vi "HFRR ADV v02.vi"() -> ()   [LabVIEW 2025] (continued)
        n289 = event-data() -> ()  [unwired: 1 in, 6 out]
        n290 = local read "Calibration"() -> (w387:bool)
        n291 = case shown="False" w387 {
          frame False {
            n292 = property on="Calibration 2" class="TabCtl (strict)"("Visible"=FALSE) -> ()  [unwired: 2 in, 2 out]
            n293 = local write "Cal Password"("" ("Cal Password")) -> ()
          }
          frame True {
            n294 = property on="Calibration 2" class="TabCtl (strict)"("Visible"=TRUE) -> ()  [unwired: 2 in, 2 out]
            n295 = local write "Cal Password"("" ("Cal Password")) -> ()
          }
        }
        n296 = property on="Wrong Password" class="Str"("Visible"=FALSE) -> ()  [unwired: 2 in, 2 out]
      }
      event "Cal Password": Value Change {
        n297 = event-data() -> ()  [unwired: 1 in, 6 out]
        n298 = local read "Cal Password"() -> (w395:string)
        n299 = call <vilib>:"Trim Whitespace.vi"("string"=w395) -> ("trimmed string"=w394:string)  [unwired: 1 in]
        n300 = Equal?(x=w394, y="Cal@321") -> (x = y?=w392:bool)
        n301 = case shown="True" w392 {
          frame False {
            n302 = property on="Wrong Password" class="Str"("Visible"=TRUE) -> ()  [unwired: 2 in, 2 out]
          }
          frame True {
            n303 = property on="Wrong Password" class="Str"("Visible"=FALSE) -> ()  [unwired: 2 in, 2 out]
            n304 = local write "Main Tab"(T2."About" ("Main Tab")) -> ()
            n305 = local write "Cal Password"("" ("Cal Password")) -> ()
            n306 = local write "Main Dashboard Buttons"(T1."About" ("Main Dashboard Buttons")) -> ()
            n307 = local write "Tab Control 5"(T7."Temperature Calibration" ("Tab Control 5")) -> ()
            n308 = property on="Calibration 2" class="TabCtl (strict)"("Visible"=FALSE) -> ()  [unwired: 2 in, 2 out]
            n309 = property on="Tab Control 5" class="TabCtl (strict)"("Tabs Visible?"=FALSE ("Page Labels Display Visible?")) -> ()  [unwired: 2 in, 2 out]
            n310 = local write "Calibration"(FALSE ("Calibration")) -> ()
          }
        }
      }
      event "Quit": Value Change {
        n311 = event-data() -> ()  [unwired: 1 in, 6 out]
      }
    }
    n312 = Wait (ms)(milliseconds to wait=u32 100) -> ()  [unwired: 1 out]
  }
  n313 = local write "Auto stop temp"(w12) -> ()
  n314 = local write "main tab sub"(enum32{"Page 1", "Page 2"}."Page 1" ("main tab sub")) -> ()
  n315 = local write "USERNAME"(w31) -> ()
  n316 = local write "Main Tab"(T2."HOME" ("Main Tab")) -> ()
  n317 = local write "USER ID"(w31) -> ()
  n318 = property on="Auto Scar Check  2" class="Clust (strict)"("Visible"=w12) -> (error out=w16:errorcluster)  [unwired: 2 in, 1 out]
  n319 = property on="Quit" class="Bool (strict)"("Value"=FALSE ("Quit")) -> (error out=w33:errorcluster)  [unwired: 2 in, 1 out]
  n320 = while {
    shift-right: [w407] -> _
    shift-left: "Enum - Selector" -> [w408]
    stop <- w409 stop-if-true
    # "Auto Start Logic Loop"
    n321 = case shown="\"close\"" w408 {
      tunnel: [w412 w418 w429 w461 w492 Auto_Start_enum."Exit" ("Enum - Selector") Auto_Start_enum."Init" ("Enum - Selector")] -> w407
      frame "Init", Default {
        n322 = local read "Auto Start Test"() -> (w411:bool)
        n323 = Select(t=Auto_Start_enum."Humidity & Temperature On" ("Enum - Selector"), s=w411, f=Auto_Start_enum."Init") -> (s? t:f=w412:T10)
      }
      frame "Humidity & Temperature On" {
        n324 = flat-sequence {
          tunnel: [Auto_Start_enum."Reach point" ("Enum - Selector")] -> w415
          frame #0 {
            w419 = T13."Disabled and Grayed Out" ("Disabled")
            w420 = TRUE ("Heater Button")
            n325 = property on="Humidity" class="Bool (strict)"("DisabledEnum"=w419) -> ()  [unwired: 2 in, 2 out]
            n326 = property on="Heater Button" class="Bool (strict)"("DisabledEnum"=w419) -> ()  [unwired: 2 in, 2 out]
            n327 = local write "Heater Button"(w420) -> ()
            n328 = local write "Humidity"(w420) -> ()
          }
          frame #1 {
            n329 = Wait (ms)(milliseconds to wait=u32 1000) -> ()  [unwired: 1 out]
          }
          frame #2 {
            w422 = TRUE ("Reach point temp")
            n330 = local write "Reach point Humidity"(w422) -> ()
            n331 = local write "Reach point temp"(w422) -> ()
          }
        }
        n332 = local read "Auto Start Test"() -> (w417:bool)
        n333 = Not(x=w417) -> (.not. x?=w416:bool)
        n334 = Select(t=Auto_Start_enum."close", s=w416, f=w415) -> (s? t:f=w418:T10)
      }
      frame "Reach point" {
        w430 = TRUE ("PAUSE")
        w438 = 1.0 ("y")
        w441 = 1.0 ("y")
        n335 = local read "Set Temperature:"() -> (w442:dbl)
        n336 = local read "Set Humidity:"() -> (w437:dbl)
        n337 = local read "Humidity ( %RH )"() -> (w443:dbl)
        n338 = Add(x=w442, y=w441) -> (x+y=w440:dbl)
        n339 = Subtract(x=w442, y=w441) -> (x-y=w439:dbl)
        n340 = Add(x=w437, y=w438) -> (x+y=w436:dbl)
        n341 = Subtract(x=w437, y=w438) -> (x-y=w435:dbl)
        n342 = local read "TEMP"() -> (w444:dbl)
        n343 = In Range and Coerce(upper limit=w436, x=w443, lower limit=w435) -> (In Range?=w424:bool)  [unwired: 1 out]
        n344 = In Range and Coerce(upper limit=w440, x=w444, lower limit=w439) -> (In Range?=w425:bool)  [unwired: 1 out]
        n345 = case shown="True" w424 {
          frame False {
          }
          frame True {
            n346 = case shown="True" "Reach point Humidity" {
              selector: "Reach point Humidity" -> [_ w450]
              frame False {
              }
              frame True {
                n347 = local read "EVENT LOG"() -> (w447:string)
                n348 = Not(x=w450) -> (.not. x?=w449:bool)
                n349 = local write "Reach point Humidity"(w449) -> ()
                n350 = call "Event Log.vi"("Content"="Target Humidity reached", "EVENT LOG"=w447) -> ("EVENT LOG"=w448:string)  [unwired: 8 in, 1 out]
                n351 = local write "EVENT LOG"(w448) -> ()
              }
            }
          }
        }
        n352 = case shown="True" w425 {
          frame False {
          }
          frame True {
            n353 = case shown="True" "Reach point temp" {
              selector: "Reach point temp" -> [_ w456]
              frame False {
              }
              frame True {
                n354 = local read "EVENT LOG"() -> (w453:string)
                n355 = Not(x=w456) -> (.not. x?=w455:bool)
                n356 = local write "Reach point temp"(w455) -> ()
                n357 = call "Event Log.vi"("Content"="Target Temperature reached", "EVENT LOG"=w453) -> ("EVENT LOG"=w454:string)  [unwired: 8 in, 1 out]
                n358 = local write "EVENT LOG"(w454) -> ()
              }
            }
          }
        }
        n359 = local read "Auto Start Test"() -> (w428:bool)
        n360 = And(x=w425, y=w424) -> (x .and. y?=w434:bool)
        n361 = Select(t=Auto_Start_enum."Maintain Stage" ("Enum - Selector"), s=w434, f=Auto_Start_enum."Reach point" ("Enum - Selector")) -> (s? t:f=w431:T10)
        n362 = Not(x=w428) -> (.not. x?=w427:bool)
        n363 = Select(t=Auto_Start_enum."close", s=w427, f=w431) -> (s? t:f=w429:T10)
        n364 = call "ELAPSED TIMER VI.vi"("RESET"=w430, "PAUSE"=w430) -> ()  [unwired: 7 in, 3 out]
      }
      frame "Maintain Stage" {
        w470 = 2.0 ("y")
        w469 = 1.0 ("y")
        # "Humidity and  temperatures Set Point  have been reached"
        n365 = local read "Set Temperature:"() -> (w476:dbl)
        n366 = local read "Set Humidity:"() -> (w473:dbl)
        n367 = local read "Humidity ( %RH )"() -> (w477:dbl)
        n368 = Add(x=w476, y=w469) -> (x+y=w475:dbl)
        n369 = Subtract(x=w476, y=w469) -> (x-y=w474:dbl)
        n370 = local read "TEMP"() -> (w478:dbl)
        n371 = Add(x=w473, y=w470) -> (x+y=w472:dbl)
        n372 = Subtract(x=w473, y=w470) -> (x-y=w471:dbl)
        n373 = In Range and Coerce(upper limit=w475, x=w478, lower limit=w474) -> (In Range?=w468:bool)  [unwired: 1 out]
        n374 = In Range and Coerce(upper limit=w472, x=w477, lower limit=w471) -> (In Range?=w467:bool)  [unwired: 1 out]
        n375 = And(x=w468, y=w467) -> (x .and. y?=w466:bool)
        n376 = Not(x=w466) -> (.not. x?=w465:bool)
        n377 = call "ELAPSED TIMER VI.vi"("TARGET"=60.0, "RESET"=w465, "PAUSE"=FALSE) -> ("ELAPSED INDICATION"=w462:bool)  [unwired: 6 in, 2 out]
        n378 = case shown="True" w462 {
          tunnel: w462 -> [_ w481]
          tunnel: [Auto_Start_enum."Maintain Stage" ("Enum - Selector") w480] -> w460
          frame False {
          }
          frame True {
            n379 = stacked-sequence {
              tunnel: w481 -> [_ _ _ _ _]
              tunnel: [_ _ _ _ Auto_Start_enum."Start Stage" ("Enum - Selector")] -> w480
              frame #0 {
                n380 = local read "EVENT LOG"() -> (w483:string)
                n381 = call "Event Log.vi"("Content"="Humidity and temperature set point has stabilized.", "EVENT LOG"=w483) -> ("EVENT LOG"=w484:string)  [unwired: 8 in, 1 out]
                n382 = local write "EVENT LOG"(w484) -> ()
              }
              frame #1 {
                n383 = Wait (ms)(milliseconds to wait=u32 100) -> ()  [unwired: 1 out]
              }
              frame #2 {
                n384 = local read "EVENT LOG"() -> (w487:string)
                n385 = call "Event Log.vi"("Content"="Auto Test Started", "EVENT LOG"=w487) -> ("EVENT LOG"=w488:string)  [unwired: 8 in, 1 out]
                n386 = local write "EVENT LOG"(w488) -> ()
              }
              frame #3 {
                w489 = TRUE ("RUN")
                n387 = local write "RUN"(w489) -> ()
                "Auto Start Temp" <- w489
              }
              frame #4 {
              }
            }
          }
        }
        n388 = local read "Auto Start Test"() -> (w459:bool)
        n389 = Not(x=w459) -> (.not. x?=w458:bool)
        n390 = Select(t=Auto_Start_enum."close", s=w458, f=w460) -> (s? t:f=w461:T10)
      }
      frame "Start Stage" {
        w491 = TRUE ("PAUSE")
        n391 = local read "Auto Start Test"() -> (w496:bool)
        n392 = Not(x=w496) -> (.not. x?=w495:bool)
        n393 = Select(t=Auto_Start_enum."close" ("Enum - Selector"), s=w495, f=Auto_Start_enum."Start Stage" ("Enum - Selector")) -> (s? t:f=w492:T10)
        n394 = call "ELAPSED TIMER VI.vi"("RESET"=w491, "PAUSE"=w491) -> ()  [unwired: 7 in, 3 out]
      }
      frame "close" {
        w497 = FALSE ("Heater Button")
        n395 = local write "RUN"(w497) -> ()
        n396 = local write "Heater Button"(w497) -> ()
        n397 = local write "Humidity"(w497) -> ()
        n398 = local write "Auto Start Test"(w497) -> ()
      }
      frame "Exit" {
      }
    }
    n399 = Wait (ms)(milliseconds to wait=u32 100) -> ()  [unwired: 1 out]
    n400 = local read "Quit"() -> (w409:bool)
  }
  n401 = while {
    stop <- w526 stop-if-true
    w509 = errorcluster {"status"=FALSE, "code"=0, "source"=""} ("error in (no error) 3")
    # "this loop is for manual report generation"
    n402 = local read "Confirm Measrurement"() -> (w508:bool)
    n403 = case shown="True" w508 {
      selector: w508 -> [_ w616]
      tunnel: errorcluster {"status"=FALSE, "code"=0, "source"=""} ("error in (no error) 3") -> [_ w617]
      tunnel: [_ w615] -> _
      frame False {
      }
      frame True {
        n404 = stacked-sequence {
          tunnel: w617 -> [_ w650 _]
          tunnel: w616 -> [_ _ w757]
          tunnel: [_ w638 _] -> w615
          frame #0 {
            n405 = String To Path(string="C:\\LAB-IQ\\Image Calibrate v01.dcf") -> (path=w620:path)
            n406 = Open/Create/Replace File ("Open File")(file path (use dialog)=w620) -> (refnum out=w621:refnum<file>)  [unwired: 5 in, 2 out]
            n407 = for {
              N: 4 -> [_]
              tunnel: w621 -> [w627]
              i -> [w623]
              n408 = Read from Text File ("Read File")(file (use dialog)=w627) -> (text=w628:string)  [unwired: 3 in, 3 out]
              n409 = String Subset(string=w628, offset (0)=6, length (rest)=10 ("length (rest)")) -> (substring=w624:string)
              n410 = Fract/Exp String To Number(string=w624) -> (number=w622:dbl)  [unwired: 3 in, 1 out]
              n411 = case shown="3" w623 {
                tunnel: w622 -> [w629 w630 _ w631 _]
                frame 0 {
                  n412 = local write "5x Gain"(w629) -> ()
                }
                frame 1 {
                  n413 = local write "10x Gain"(w630) -> ()
                }
                frame 2 {
                }
                frame 3 {
                  n414 = local write "100x gain"(w631) -> ()
                }
                frame 4, Default {
                }
              }
            }
          }
          frame #1 {
            n415 = local read "TEST STANDARD"() -> (w633:T3)
            n416 = case shown="\"ISO 12156\"" w633 {
              tunnel: ["ASTM D6079" "ISO 12156"] -> w632
              frame "ASTM D6079", Default {
              }
              frame "ISO 12156" {
              }
            }
            n417 = call "IMAGE ANALYSIS.vi"("Enum"=POST_ANALYSIS_ENUM."GET MEASUREMENTS", "error in"=w650) -> ("error out"=w657:errorcluster)  [unwired: 8 in, 1 out]
            n418 = local read "Magnification :"() -> (w643:string)
            n419 = call "Stall Data Flow.vim"("value in"=w657, "milliseconds to wait"=u32 1000) -> ("value out"=w656:errorcluster)  [unwired: 1 out]
            n420 = local read "Test File List :"() -> (w654:string)
            n421 = case shown="\"10x\"" w643 {
              tunnel: [w693 w694] -> w641
              frame "5x", Default {
                n422 = local read "5x Gain"() -> (w693:dbl)
              }
              frame "10x" {
                # "5x"
                n423 = local read "10x Gain"() -> (w694:dbl)
              }
            }
            n424 = call "IMAGE ANALYSIS.vi"("Enum"=POST_ANALYSIS_ENUM."READ", "error in"=w656) -> ("error out"=w653:errorcluster, "data out"=w644:string)  [unwired: 8 in]
            n425 = Match Pattern(string=w644, regular expression="\"type\": ") -> (after substring=w648:string)  [unwired: 1 in, 3 out]
            n426 = call "IMAGE PATH CREATION PY.vi"("error in (no error)"=w653, "File Name :"=w654) -> ("error out"=w652:errorcluster, "File Path"=w640:path, "File Path String:"=w635:string)  [unwired: 7 in]
            n427 = Match Pattern(string=w648, regular expression=",") -> (before substring=w634:string)  [unwired: 1 in, 3 out]
            n428 = local read "Calibration Tab"() -> (w637:enum32{"Measrument", "Calibrate"})
            n429 = call "Stall Data Flow.vim"("value in"=w652, "milliseconds to wait"=u32 250) -> ("value out"=w636:errorcluster)  [unwired: 1 out]
            n430 = Equal?(x=w634, y="\"rectangle\"") -> (x = y?=w645:bool)
            n431 = case shown="False" w645 {
              tunnel: w644 -> [w699 w754]
              tunnel: w641 -> [_ w745]
              tunnel: cluster{"major":dbl, "minor":dbl, "average":dbl} {"major"=0.0, "minor"=0.0, "average"=0.0} -> [w697 w741]
              tunnel: [w696 w738] -> w639
              tunnel: w634 -> [w698 _]
              tunnel: w641 -> [w695 _]
              frame False {
                n432 = Equal?(x=w698, y="\"line\"") -> (x = y?=w700:bool)
                n433 = case shown="True" w700 {
                  tunnel: w699 -> [_ w715]
                  tunnel: w697 -> [w702 w714]
                  tunnel: [w702 w712] -> w696
                  tunnel: w695 -> [_ w711]
                  frame False {
                  }
                  frame True {
                    w710 = 0.0 ("Major Axis")
                    n434 = Match Pattern(string=w715, regular expression="\"length_px\":") -> (after substring=w713:string)  [unwired: 1 in, 3 out]
                    n435 = property on="Major Axis" class="DigNum (strict)"("Caption.Text"="") -> ()  [unwired: 2 in, 2 out]
                    n436 = property on="Minor Axis" class="DigNum (strict)"("Caption.Text"="") -> ()  [unwired: 2 in, 2 out]
                    n437 = property on="Average" class="DigNum (strict)"("Caption.Text"="Line") -> ()  [unwired: 2 in, 2 out]
                    n438 = Fract/Exp String To Number(string=w713, default (0 dbl)=0.0 ("default (0 DBL)")) -> (number=w709:dbl)  [unwired: 2 in, 1 out]
                    "Pixel Value" <- w709
                    n439 = Multiply(x=w709, y=w711) -> (x*y=w722:dbl)
                    n440 = Multiply(x=w722, y=1000.0) -> (x*y=w705:dbl)
                    n441 = Divide(x=w705, y=1000.0) -> (x/y=w708:dbl)
                    n442 = local write "Measurment (mm)"(w708) -> ()
                    n443 = Bundle By Name(cluster=w714, "average"=w705) -> (w712:cluster{"major":dbl, "minor":dbl, "average":dbl})
                    n444 = Number To Fractional String(number=w705, precision (6)=i16 1) -> (F-format string=w704:string)  [unwired: 2 in]
                    n445 = local write "Minor Axis"(w710) -> ()
                    n446 = local write "Major Axis"(w710) -> ()
                    n447 = Fract/Exp String To Number(string=w704) -> (number=w703:dbl)  [unwired: 3 in, 1 out]
                    n448 = local write "Average"(w703) -> ()
                  }
                }
              }
              frame True {
                w742 = 1000.0 ("y")
                w748 = 0.0 ("default (0 DBL)")
                n449 = Match Pattern(string=w754, regular expression=" \"width_px\":") -> (after substring=w752:string)  [unwired: 1 in, 3 out]
                n450 = Match Pattern(string=w752, regular expression="\"height_px\":") -> (before substring=w750:string, after substring=w749:string)  [unwired: 1 in, 2 out]
                n451 = Fract/Exp String To Number(string=w750, default (0 dbl)=w748) -> (number=w747:dbl)  [unwired: 2 in, 1 out]
                n452 = Fract/Exp String To Number(string=w749, default (0 dbl)=w748) -> (number=w746:dbl)  [unwired: 2 in, 1 out]
                n453 = Multiply(x=w747, y=w745) -> (x*y=w744:dbl)
                n454 = Multiply(x=w746, y=w745) -> (x*y=w743:dbl)
                n455 = Multiply(x=w744, y=w742) -> (x*y=w728:dbl)
                n456 = Multiply(x=w743, y=w742) -> (x*y=w726:dbl)
                n457 = Add(x=w728, y=w726) -> (x+y=w740:dbl)
                n458 = property on="Major Axis" class="DigNum (strict)"("Caption.Text"="Major Axis") -> ()  [unwired: 2 in, 2 out]
                n459 = property on="Minor Axis" class="DigNum (strict)"("Caption.Text"="Minor Axis") -> ()  [unwired: 2 in, 2 out]
                n460 = property on="Average" class="DigNum (strict)"("Caption.Text"="Average") -> ()  [unwired: 2 in, 2 out]
                n461 = Divide(x=w740, y=2.0) -> (x/y=w724:dbl)
                n462 = Bundle By Name(cluster=w741, "major"=w728, "minor"=w726, "average"=w724) -> (w738:cluster{"major":dbl, "minor":dbl, "average":dbl})
                n463 = Number To Fractional String(number=w726, precision (6)=i16 1) -> (F-format string=w733:string)  [unwired: 2 in]
                n464 = Number To Fractional String(number=w724, precision (6)=i16 1) -> (F-format string=w734:string)  [unwired: 2 in]
                n465 = Number To Fractional String(number=w728, precision (6)=i16 1) -> (F-format string=w732:string)  [unwired: 2 in]
                n466 = Fract/Exp String To Number(string=w733) -> (number=w725:dbl)  [unwired: 3 in, 1 out]
                n467 = Fract/Exp String To Number(string=w734) -> (number=w723:dbl)  [unwired: 3 in, 1 out]
                n468 = Fract/Exp String To Number(string=w732) -> (number=w727:dbl)  [unwired: 3 in, 1 out]
                n469 = local write "Major Axis"(w727) -> ()
                n470 = local write "Average"(w723) -> ()
                n471 = local write "Minor Axis"(w725) -> ()
              }
            }
            n472 = case shown="\"Measrument\", Default" w637 {
              tunnel: w640 -> [w667 _]
              tunnel: w639 -> [w666 _]
              tunnel: [w663 w692] -> w638
              tunnel: w636 -> [w665 w692]
              tunnel: w635 -> [w664 _]
              tunnel: w632 -> [w662 _]
              frame "Measrument", Default {
                n473 = stacked-sequence {
                  tunnel: w667 -> [w685 _]
                  tunnel: w666 -> [w683 _]
                  tunnel: w665 -> [w681 _]
                  tunnel: w664 -> [w680 _]
                  tunnel: [w675 _] -> w663
                  tunnel: w662 -> [w668 _]
                  frame #0 {
                    n474 = call "IMAGE ANALYSIS.vi"("Enum"=POST_ANALYSIS_ENUM."SAVE IMAGE", "error in"=w681, "IMAGE FILE PATH"=w680) -> ("error out"=w679:errorcluster)  [unwired: 7 in, 1 out]
                    n475 = call "Stall Data Flow.vim"("value in"=w679, "milliseconds to wait"=u32 1000) -> ("value out"=w670:errorcluster)  [unwired: 1 out]
                    n476 = local read "Test File List :"() -> (w687:string)
                    n477 = call "IMAGE ANALYSIS.vi"("Enum"=POST_ANALYSIS_ENUM."MINIMIZE UI", "error in"=w670) -> ("error out"=w677:errorcluster)  [unwired: 8 in, 1 out]
                    n478 = Bundle By Name(cluster=T18 {"File Name"="", "Test Method"="", "Operator"="", "Fuel Description"="", "Date and time"=""} ("Main Ref"), "Test Method"=w668, "File Name"=w687) -> (w688:T18)
                    n479 = call "Stall Data Flow.vim"("value in"=w677, "milliseconds to wait"=u32 1500) -> ("value out"=w672:errorcluster)  [unwired: 1 out]
                    n480 = call "duf file read.vi"("error in (no error)"=w672, "Main Ref"=w688) -> ("error out"=w686:errorcluster, "Main Ref 2"=w684:T18)  [unwired: 8 in]
                    n481 = call "DETECTION REPORT for manual.vi"("error in (no error)"=w686, "return value 3"=w683, "Image File Path"=w685, "Main Ref"=w684) -> ("error out"=w682:errorcluster)  [unwired: 7 in]
                    n482 = call <vilib>:"Clear Errors.vi"("error in (no error)"=w682) -> ("error out"=w673:errorcluster)  [unwired: 5 in, 1 out]
                    n483 = call "IMAGE ANALYSIS.vi"("Enum"=POST_ANALYSIS_ENUM."MINIMIZE UI", "error in"=w673) -> ("error out"=w675:errorcluster)  [unwired: 8 in, 1 out]
                  }
                  frame #1 {
                    n484 = local write "Main Tab"(T2."HOME" ("Main Tab")) -> ()
                    n485 = local write "Main Dashboard Buttons"(T1."Home" ("Main Dashboard Buttons")) -> ()
                  }
                }
              }
              frame "Calibrate" {
              }
            }
          }
          frame #2 {
            n486 = Not(x=w757) -> (.not. x?=w756:bool)
            n487 = local write "Confirm Measrurement"(w756) -> ()
            n488 = local read "Calibration Tab"() -> (w755:enum32{"Measrument", "Calibrate"})
            n489 = case shown="\"Measrument\", Default" w755 {
              frame "Measrument", Default {
                n490 = local write "Main Tab"(T2."HOME" ("Main Tab")) -> ()
              }
              frame "Calibrate" {
              }
            }
          }
        }
      }
    }
    n491 = local read "Humidity"() -> (w500:bool)
    n492 = local read "Save Change"() -> (w505:bool)
    n493 = local read "Calibrate"() -> (w506:bool)
    n494 = local read "Auto Start Test"() -> (w501:bool)
    n495 = case shown="True" w506 {
      selector: w506 -> [_ w613]
      frame False {
      }
      frame True {
        n496 = Not(x=w613) -> (.not. x?=w612:bool)
        n497 = local write "Calibrate"(w612) -> ()
        n498 = local write "Calibration Tab"(enum32{"Measrument", "Calibrate"}."Calibrate" ("Calibration Tab")) -> ()
      }
    }
    n499 = case shown="True" w505 {
      selector: w505 -> [_ w557]
      frame False {
      }
      frame True {
        n500 = stacked-sequence {
          tunnel: w557 -> [_ _ _ _ w611]
          frame #0 {
            n501 = call "IMAGE ANALYSIS.vi"("Enum"=POST_ANALYSIS_ENUM."HIDE UI") -> ()  [unwired: 9 in, 2 out]
          }
          frame #1 {
            n502 = local read "100x gain"() -> (w559:dbl)
            n503 = local read "10x Gain"() -> (w560:dbl)
            n504 = local read "5x Gain"() -> (w561:dbl)
            n505 = Number To Fractional String(number=w560, width (-)=i16 4, precision (6)=i16 7) -> (F-format string=w582:string)  [unwired: 1 in]
            n506 = Number To Fractional String(number=0.0, width (-)=i16 4, precision (6)=i16 7) -> (F-format string=w577:string)  [unwired: 1 in]
            n507 = Number To Fractional String(number=w559, width (-)=i16 4, precision (6)=i16 7) -> (F-format string=w565:string)  [unwired: 1 in]
            n508 = Number To Fractional String(number=w561, width (-)=i16 10 ("precision (6)"), precision (6)=i16 7) -> (F-format string=w591:string)  [unwired: 1 in]
            n509 = Concatenate Strings("[CH1]" ("string"), w591, " - 5x Gain" ("string"), "\r") -> (w581:string)
            n510 = Concatenate Strings("[CH2]" ("string"), w582, " - 10x Gain" ("string"), "\r") -> (w580:string)
            n511 = Concatenate Strings("[CH3]" ("string"), w577, " - 20x Gain" ("string"), "\r") -> (w571:string)
            n512 = Concatenate Strings("[CH4]" ("string"), w565, " - 100x Gain" ("string"), "\r") -> (w564:string)
            n513 = String To Path(string="C:\\LAB-IQ\\Image Calibrate v01.dcf") -> (path=w594:path)
            n514 = Concatenate Strings(w581, w580, w571, w564) -> (w579:string)
            n515 = call <vilib>:"Write Characters To File.vi"("append to file? (new file:F)"=FALSE, "character string"=w579, "file path (dialog if empty)"=w594) -> ()  [unwired: 2 in, 1 out]
          }
          frame #2 {
            n516 = String To Path(string="C:\\LAB-IQ\\Image Calibrate v01.dcf") -> (path=w597:path)
            n517 = Open/Create/Replace File ("Open File")(file path (use dialog)=w597) -> (refnum out=w598:refnum<file>)  [unwired: 5 in, 2 out]
            n518 = for {
              N: 4 -> [_]
              tunnel: w598 -> [w604]
              i -> [w600]
              n519 = Read from Text File ("Read File")(file (use dialog)=w604) -> (text=w605:string)  [unwired: 3 in, 3 out]
              n520 = String Subset(string=w605, offset (0)=6, length (rest)=10 ("length (rest)")) -> (substring=w601:string)
              n521 = Fract/Exp String To Number(string=w601) -> (number=w599:dbl)  [unwired: 3 in, 1 out]
              n522 = case shown="3" w600 {
                tunnel: w599 -> [w606 w607 _ w608 _]
                frame 0 {
                  n523 = local write "5x Gain"(w606) -> ()
                }
                frame 1 {
                  n524 = local write "10x Gain"(w607) -> ()
                }
                frame 2 {
                }
                frame 3 {
                  n525 = local write "100x gain"(w608) -> ()
                }
                frame 4, Default {
                }
              }
            }
          }
          frame #3 {
            n526 = call "IMAGE ANALYSIS.vi"("Enum"=POST_ANALYSIS_ENUM."SHOW UI") -> ()  [unwired: 9 in, 2 out]
          }
          frame #4 {
            n527 = Not(x=w611) -> (.not. x?=w610:bool)
            n528 = local write "Save Change"(w610) -> ()
          }
        }
      }
    }
    n529 = case shown="False" w501 {
      tunnel: w500 -> [w527 _]
      frame False {
        n530 = case shown="True" w527 {
          frame False {
          }
          frame True {
            n531 = local read "Set Humidity:"() -> (w531:dbl)
            n532 = local read "Set Humidity:"() -> (w534:dbl)
            n533 = local read "Humidity ( %RH )"() -> (w535:dbl)
            n534 = Subtract(x=w531, y=2.0) -> (x-y=w529:dbl)
            n535 = Add(x=w534, y=2.0) -> (x+y=w530:dbl)
            n536 = In Range and Coerce(upper limit=w530, x=w535, lower limit=w529) -> (In Range?=w528:bool)  [unwired: 1 out]
            n537 = case shown="True" w528 {
              frame False {
              }
              frame True {
                n538 = case shown="False" "Manual Humididty Reached" {
                  selector: "Manual Humididty Reached" -> [_ w538]
                  frame False {
                  }
                  frame True {
                    n539 = Not(x=w538) -> (.not. x?=w537:bool)
                    n540 = local write "Manual Humididty Reached"(w537) -> ()
                    n541 = local read "EVENT LOG"() -> (w540:string)
                    n542 = call "Event Log.vi"("Content"="Target Humidity reached", "EVENT LOG"=w540) -> ("EVENT LOG"=w539:string)  [unwired: 8 in, 1 out]
                    n543 = local write "EVENT LOG"(w539) -> ()
                  }
                }
              }
            }
          }
        }
      }
      frame True {
        n544 = local write "Manual Humididty Reached"(TRUE ("Manual Humididty Reached")) -> ()
      }
    }
    n545 = local read "Cap Live Image"() -> (w521:bool)
    n546 = local read "SCAR MEASURMENT"() -> (w524:enum32{"Auto Scar", "Manual Scar"})
    n547 = Wait (ms)(milliseconds to wait=u32 250) -> ()  [unwired: 1 out]
    n548 = Equal?(x=w524, y=enum32{"Auto Scar", "Manual Scar"}."Manual Scar" ("SCAR MEASURMENT")) -> (x = y?=w522:bool)
    n549 = And(x=w522, y=w521) -> (x .and. y?=w520:bool)
    n550 = case shown="True" w520 {
      selector: w520 -> [_ w836]
      frame False {
      }
      frame True {
        n551 = stacked-sequence {
          tunnel: [_ _ _ w851 _] -> _
          tunnel: w836 -> [_ _ _ _ w857]
          frame #0 {
            w837 = 0.0
            n552 = local write "Major Axis"(w837) -> ()
            n553 = local write "Minor Axis"(w837) -> ()
            n554 = local write "Average"(w837) -> ()
          }
          frame #1 {
            n555 = call "CAMERA LIVE FEED FGV.vi"("Enum - Menu"=CAMERA_LIVE_FEED_ENUM."CAMERA MINIMIZE") -> ()  [unwired: 9 in, 2 out]
          }
          frame #2 {
            n556 = local read "FILE 3"() -> (w845:string)
            n557 = call <vilib>:"Trim Whitespace.vi"("string"="C:\\LAB-IQ\\images\\") -> ("trimmed string"=w847:string)  [unwired: 1 in]
            n558 = String To Path(string=w847) -> (path=w846:path)
            n559 = Concatenate Strings(w845, ".png" ("string")) -> (w844:string)
            n560 = Build Path(base path=w846, name or relative path=w844) -> (appended path=w842:path)
            n561 = Path To String(path=w842) -> (string=w841:string)
            n562 = call "CAMERA LIVE FEED FGV.vi"("Enum - Menu"=CAMERA_LIVE_FEED_ENUM."CAMERA SAVE", "Image Path"=w841) -> ("error out"=w839:errorcluster)  [unwired: 8 in, 1 out]
            n563 = case shown="No Error" w839 {
              frame No Error {
                n564 = One Button Dialog(message="Image saved successfully") -> ()  [unwired: 1 in, 1 out]
              }
              frame Error {
              }
            }
          }
          frame #3 {
            n565 = call "LIST FILE NAMES.vi"() -> ("error out"=w853:errorcluster, "filenames"=w850:string[])  [unwired: 10 in]
            n566 = call "IMAGE ANALYSIS.vi"("Enum"=POST_ANALYSIS_ENUM."SHOW UI", "error in"=w853) -> ("error out"=w851:errorcluster)  [unwired: 8 in, 1 out]
            n567 = property on="Test File List :" class="CmbBox"("Strings[]"=w850) -> ()  [unwired: 2 in, 2 out]
          }
          frame #4 {
            (unwired) T19."Report" ("Main Dashboard Buttons")
            n568 = Not(x=w857) -> (.not. x?=w856:bool)
            n569 = local write "Zoom Factore"(0.0 ("Zoom Factore")) -> ()
            n570 = local write "Cap Live Image"(w856) -> ()
            n571 = local write "Main Tab"(T2."Adv Scar Report" ("Main Tab")) -> ()
            n572 = property on="Cap Live Image" class="Bool (strict)"("BoolText.Text"="Capture Image" ("Boolean Text.Text")) -> ()  [unwired: 2 in, 2 out]
            n573 = local write "Main Dashboard Buttons"(T1."Report" ("Main Dashboard Buttons")) -> ()
          }
        }
      }
    }
    n574 = local read "change Gain"() -> (w504:bool)
    n575 = local read "Back Square"() -> (w503:bool)
    n576 = case shown="True" w504 {
      selector: w504 -> [_ w548]
      frame False {
      }
      frame True {
        n577 = stacked-sequence {
          tunnel: w548 -> [_ w556]
          frame #0 {
            n578 = local read "Actual (µm)"() -> (w552:dbl)
            n579 = local read "Pixel Value"() -> (w551:dbl)
            n580 = local read "Magnification :"() -> (w550:string)
            n581 = Divide(x=w552, y=w551) -> (x/y=w549:dbl)
            n582 = case shown="\"10x\"" w550 {
              tunnel: w549 -> [w553 w554]
              frame "10x" {
                n583 = local write "10x Gain"(w553) -> ()
              }
              frame "5x", Default {
                n584 = local write "5x Gain"(w554) -> ()
              }
            }
          }
          frame #1 {
            n585 = Not(x=w556) -> (.not. x?=w555:bool)
            n586 = local write "change Gain"(w555) -> ()
          }
        }
      }
    }
    n587 = case shown="True" w503 {
      selector: w503 -> [_ w546]
      frame False {
      }
      frame True {
        n588 = Not(x=w546) -> (.not. x?=w545:bool)
        n589 = local write "Back Square"(w545) -> ()
        n590 = local write "Calibration Tab"(enum32{"Measrument", "Calibrate"}."Measrument" ("Calibration Tab")) -> ()
      }
    }
    n591 = local read "Rectangle Tool"() -> (w515:bool)
    n592 = local read "Clear ROI Tool"() -> (w514:bool)
    n593 = local read "Open Image"() -> (w519:bool)
    n594 = local read "line tool"() -> (w516:bool)
    n595 = local read "OUT"() -> (w517:bool)
    n596 = local read "In"() -> (w518:bool)
    n597 = case shown="True" w519 {
      selector: w519 -> [_ w824]
      tunnel: [w820 w826] -> _
      tunnel: w509 -> [w820 w825]
      frame False {
      }
      frame True {
        n598 = Not(x=w824) -> (.not. x?=w823:bool)
        n599 = local write "Open Image"(w823) -> ()
        n600 = call "IMAGE ANALYSIS.vi"("Enum"=POST_ANALYSIS_ENUM."HIDE UI", "error in"=w825) -> ("error out"=w833:errorcluster)  [unwired: 8 in, 1 out]
        n601 = call "File Dialog"("start path"=path "C:/LAB-IQ/images", "error in"=w833) -> ("selected path"=w822:path, "error out"=w831:errorcluster)  [unwired: 10 in, 2 out]
        "Image path  2" <- w822
        n602 = call <vilib>:"Clear Errors.vi"("error in (no error)"=w831) -> ("error out"=w830:errorcluster)  [unwired: 5 in, 1 out]
        n603 = call "IMAGE ANALYSIS.vi"("Enum"=POST_ANALYSIS_ENUM."OPEN FILE", "error in"=w830, "File Path"=w822) -> ("error out"=w829:errorcluster)  [unwired: 7 in, 1 out]
        n604 = call <vilib>:"Clear Errors.vi"("error in (no error)"=w829) -> ("error out"=w828:errorcluster)  [unwired: 5 in, 1 out]
        n605 = call "IMAGE ANALYSIS.vi"("Enum"=POST_ANALYSIS_ENUM."SHOW UI", "error in"=w828) -> ("error out"=w826:errorcluster)  [unwired: 8 in, 1 out]
        n606 = local write "Zoom Factore"(100.0 ("Zoom Factore")) -> ()
      }
    }
    n607 = case shown="True" w517 {
      selector: w517 -> [_ w805]
      tunnel: w509 -> [w802 w810]
      tunnel: [w802 w804] -> _
      frame False {
      }
      frame True {
        n608 = Not(x=w805) -> (.not. x?=w803:bool)
        n609 = local read "Zoom Factore"() -> (w808:dbl)
        n610 = local write "OUT"(w803) -> ()
        n611 = call "IMAGE ANALYSIS.vi"("Enum"=POST_ANALYSIS_ENUM."ZOOM OUT", "error in"=w810) -> ("error out"=w804:errorcluster)  [unwired: 8 in, 1 out]
        n612 = Divide(x=w808, y=1.2) -> (x/y=w806:dbl)
        n613 = local write "Zoom Factore"(w806) -> ()
      }
    }
    n614 = case shown="True" w518 {
      selector: w518 -> [_ w814]
      tunnel: w509 -> [w811 w819]
      tunnel: [w811 w812] -> _
      frame False {
      }
      frame True {
        n615 = Not(x=w814) -> (.not. x?=w813:bool)
        n616 = local read "Zoom Factore"() -> (w817:dbl)
        n617 = local write "In"(w813) -> ()
        n618 = call "IMAGE ANALYSIS.vi"("Enum"=POST_ANALYSIS_ENUM."ZOOM IN", "error in"=w819) -> ("error out"=w812:errorcluster)  [unwired: 8 in, 1 out]
        n619 = Multiply(x=w817, y=1.2) -> (x*y=w815:dbl)
        n620 = local write "Zoom Factore"(w815) -> ()
      }
    }
    n621 = case shown="True" w514 {
      selector: w514 -> [_ w786]
      tunnel: w509 -> [w784 w788]
      tunnel: [w784 w787] -> _
      frame False {
      }
      frame True {
        n622 = Not(x=w786) -> (.not. x?=w785:bool)
        n623 = local write "Clear ROI Tool"(w785) -> ()
        n624 = call "IMAGE ANALYSIS.vi"("Enum"=POST_ANALYSIS_ENUM."CLEAR ROI", "error in"=w788) -> ("error out"=w787:errorcluster)  [unwired: 8 in, 1 out]
      }
    }
    n625 = case shown="True" w516 {
      selector: w516 -> [_ w798]
      tunnel: w509 -> [w796 w801]
      tunnel: [w796 w799] -> _
      frame False {
      }
      frame True {
        n626 = Not(x=w798) -> (.not. x?=w797:bool)
        n627 = local write "line tool"(w797) -> ()
        n628 = call "IMAGE ANALYSIS.vi"("Enum"=POST_ANALYSIS_ENUM."DRAW LINE", "error in"=w801) -> ("error out"=w799:errorcluster)  [unwired: 8 in, 1 out]
      }
    }
    n629 = case shown="True" w515 {
      selector: w515 -> [_ w792]
      tunnel: w509 -> [w790 w794]
      tunnel: [w790 w793] -> _
      frame False {
      }
      frame True {
        n630 = Not(x=w792) -> (.not. x?=w791:bool)
        n631 = local write "Rectangle Tool"(w791) -> ()
        n632 = call "IMAGE ANALYSIS.vi"("Enum"=POST_ANALYSIS_ENUM."DRAW REC", "error in"=w794) -> ("error out"=w793:errorcluster)  [unwired: 8 in, 1 out]
      }
    }
    n633 = local read "SCAR MEASURMENT"() -> (w502:enum32{"Auto Scar", "Manual Scar"})
    n634 = local read "Fit to Screen Tool"() -> (w511:bool)
    n635 = local read "Resize Tool"() -> (w510:bool)
    n636 = case shown="\"Manual Scar\", Default" w502 {
      frame "Auto Scar" {
        n637 = property on="Cap Live Image" class="Bool (strict)"("BoolText.Text"="Report" ("Boolean Text.Text")) -> ()  [unwired: 2 in, 2 out]
      }
      frame "Manual Scar", Default {
        n638 = property on="Cap Live Image" class="Bool (strict)"("BoolText.Text"="Save Image" ("Boolean Text.Text")) -> ()  [unwired: 2 in, 2 out]
      }
    }
    n639 = local read "ROI Color Tool"() -> (w512:bool)
    n640 = local read "Pan Tool"() -> (w513:bool)
    n641 = case shown="True" w513 {
      selector: w513 -> [_ w780]
      tunnel: w509 -> [w778 w782]
      tunnel: [w778 w781] -> _
      frame False {
      }
      frame True {
        n642 = Not(x=w780) -> (.not. x?=w779:bool)
        n643 = call "IMAGE ANALYSIS.vi"("Enum"=POST_ANALYSIS_ENUM."PAN", "error in"=w782) -> ("error out"=w781:errorcluster)  [unwired: 8 in, 1 out]
        n644 = local write "Pan Tool"(w779) -> ()
      }
    }
    n645 = case shown="True" w510 {
      selector: w510 -> [_ w764]
      tunnel: w509 -> [w759 w761]
      tunnel: [w759 w760] -> _
      frame False {
      }
      frame True {
        n646 = Not(x=w764) -> (.not. x?=w763:bool)
        n647 = local write "Resize Tool"(w763) -> ()
        n648 = call "IMAGE ANALYSIS.vi"("Enum"=POST_ANALYSIS_ENUM."RESIZE MODE", "error in"=w761) -> ("error out"=w760:errorcluster)  [unwired: 8 in, 1 out]
      }
    }
    n649 = case shown="True" w511 {
      selector: w511 -> [_ w769]
      tunnel: [w765 w770] -> _
      tunnel: w509 -> [w765 w768]
      frame False {
      }
      frame True {
        n650 = Not(x=w769) -> (.not. x?=w767:bool)
        n651 = local write "Zoom Factore"(100.0 ("Zoom Factore")) -> ()
        n652 = local write "Fit to Screen Tool"(w767) -> ()
        n653 = call "IMAGE ANALYSIS.vi"("Enum"=POST_ANALYSIS_ENUM."FIT", "error in"=w768) -> ("error out"=w770:errorcluster)  [unwired: 8 in, 1 out]
      }
    }
    n654 = case shown="True" w512 {
      selector: w512 -> [_ w775]
      tunnel: [w772 w776] -> _
      tunnel: w509 -> [w772 w773]
      frame False {
      }
      frame True {
        n655 = Not(x=w775) -> (.not. x?=w774:bool)
        n656 = local write "ROI Color Tool"(w774) -> ()
        n657 = call "IMAGE ANALYSIS.vi"("Enum"=POST_ANALYSIS_ENUM."SET ROI COLOR", "error in"=w773) -> ("error out"=w776:errorcluster)  [unwired: 8 in, 1 out]
      }
    }
    n658 = local read "Quit"() -> (w526:bool)
  }
  n659 = while {
    stop <- w860 stop-if-true
    n660 = local read "Image Path"() -> (w863:path)
    n661 = local read "Print 3"() -> (w866:bool)
    n662 = Equal?(x=w863, y=path "") -> (x = y?=w862:bool)
    n663 = Not(x=w862) -> (.not. x?=w861:bool)
    n664 = property on="Print 3" class="Bool (strict)"("Visible"=w861) -> ()  [unwired: 2 in, 2 out]
    n665 = case shown="True" w866 {
      frame False {
        n666 = local write "Rd"(TRUE ("Boolean 7")) -> ()
      }
      frame True {
        n667 = flat-sequence {
          tunnel: [w906] -> w874
          tunnel: [w893] -> w872
          tunnel: [w903] -> w868
          tunnel: w874 -> [w915]
          tunnel: [w915] -> w873
          tunnel: w872 -> [w914]
          tunnel: [w914] -> w871
          tunnel: [w912] -> w870
          tunnel: [w911] -> w869
          tunnel: w868 -> [w911]
          tunnel: w873 -> [w917]
          tunnel: w871 -> [w918]
          tunnel: w870 -> [_]
          tunnel: w869 -> [w916]
          frame #0 {
            n668 = case shown="True" "Rd" {
              frame False {
              }
              frame True {
                n669 = while {
                  tunnel: "abcdefABCDEF" ("string 2") -> [w885]
                  shift-right: [w883] -> w877
                  shift-left: "" -> [w882]
                  i -> [w892]
                  stop <- w891 stop-if-true
                  n670 = Random Number (0-1)() -> (number: 0 to 1=w886:dbl)
                  n671 = Multiply(x=w886, y=62.0) -> (x*y=w888:dbl)
                  n672 = Decrement(x="Length 2") -> (x-1=w881:i16)
                  n673 = To Word Integer(number=w888) -> (16bit integer=w889:i16)
                  n674 = String Subset(string=w885, offset (0)=w889, length (rest)=1 ("length (rest)")) -> (substring=w884:string)
                  n675 = Greater Or Equal?(x=w892, y=w881) -> (x >= y?=w891:bool)
                  n676 = Concatenate Strings(w884, w882) -> (w883:string)
                }
                "String 10" <- w877
                n677 = local write "Rd"(FALSE ("Boolean 7")) -> ()
              }
            }
          }
          frame #1 {
            w904 = "_resized.jpg" ("command line")
            (unwired) ".jpg -resize 320x240 " ("string")
            (unwired) "Choose an Image File" ("prompt")
            # "-resize 1798x425"
            n678 = local read "Image Path"() -> (w898:path)
            n679 = Strip Path(path=w898) -> (stripped path=w893:path, name=w894:string)
            n680 = Match Pattern(string=w894, regular expression=".jpg") -> (before substring=→"before substring 2":string, after substring=→"after substring":string)  [unwired: 1 in, 2 out]
            n681 = Match Pattern(string=w894, regular expression="\\") -> (before substring=w900:string)  [unwired: 1 in, 3 out]
            n682 = Match Pattern(string=w900, regular expression=".jpg") -> (before substring=w899:string)  [unwired: 1 in, 3 out]
            n683 = Concatenate Strings("cmd /c convert " ("string"), w899, ".jpg -resize 320x240  " ("command line"), w899, w904) -> (w907:string)
            n684 = call <vilib>:"System Exec.vi"("run minimized? (F)"=TRUE, "wait until completion? (T)"=TRUE, "working directory"=w893, "command line"=w907) -> ("error out"=w906:errorcluster)  [unwired: 4 in, 3 out]
            "error out 2" <- w906
            n685 = Concatenate Strings(w899, w904) -> (w903:string)
          }
          frame #2 {
            n686 = Wait (ms)(milliseconds to wait=u32 2000 ("millisecond timer value")) -> (millisecond timer value=w912:u32)
          }
          frame #3 {
            n687 = case shown="No Error" w917 {
              tunnel: w918 -> [w921 _]
              tunnel: w916 -> [w919 _]
              frame No Error {
                (unwired) ".jpg" ("string")
                n688 = Path To String(path=w921) -> (string=w925:string)
                n689 = Concatenate Strings(w925, "\\" ("string"), w919) -> (w924:string)
                n690 = String To Path(string=w924) -> (path=w923:path)
                n691 = call <vilib>:"Read JPEG File.vi"("path to JPEG file"=w923) -> ("image data"=w927:T11)  [unwired: 8 in, 2 out]
                "image data" <- w927
                n692 = local write "Print 3"(FALSE ("Print 2")) -> ()
                n693 = call <vilib>:"Draw Flattened Pixmap.vi"("image data"=w927) -> ("new picture"=→"new picture":picture)  [unwired: 8 in]
              }
              frame Error {
              }
            }
          }
        }
      }
    }
    n694 = Wait (ms)(milliseconds to wait=u32 20 ("millisecond timer value")) -> ()  [unwired: 1 out]
    n695 = local read "Quit"() -> (w860:bool)
  }
  n696 = property on="Service Password Log" class="Str"("Visible"=w12) -> ()  [unwired: 2 in, 2 out]
  n697 = property on="Password 3" class="Clust (strict)"("Visible"=w12) -> ()  [unwired: 2 in, 2 out]
  n698 = while {
    tunnel: w33 -> [_]
    tunnel: w16 -> [_]
    stop <- w958 stop-if-true
    # "New Adv Logics"
    n699 = local read "Main Tab"() -> (w937:T2)
    n700 = local read "Main Tab"() -> (w956:T2)
    n701 = local read "Sign In"() -> (w955:bool)
    n702 = case shown="\"Adv Scar\"" w937 {
      frame "HOME", Default {
        n703 = local read "LIVE FEED MIN TEMP"() -> (w1085:bool)
        n704 = local write "LIVE FEED MAX TEMP"(TRUE ("LIVE FEED MAX TEMP")) -> ()
        n705 = local read "CAMERA ROI MIN TEMP"() -> (w1083:bool)
        n706 = case shown="True" w1085 {
          selector: w1085 -> [_ w1092]
          frame False {
          }
          frame True {
            n707 = Not(x=w1092) -> (.not. x?=w1091:bool)
            n708 = local write "LIVE FEED MIN TEMP"(w1091) -> ()
            n709 = call "CAMERA LIVE FEED FGV.vi"("Enum - Menu"=CAMERA_LIVE_FEED_ENUM."CAMERA MINIMIZE") -> ()  [unwired: 9 in, 2 out]
          }
        }
        n710 = case shown="True" w1083 {
          selector: w1083 -> [_ w1089]
          frame False {
          }
          frame True {
            n711 = Not(x=w1089) -> (.not. x?=w1088:bool)
            n712 = local write "CAMERA ROI MIN TEMP"(w1088) -> ()
            n713 = call "IMAGE ANALYSIS.vi"("Enum"=POST_ANALYSIS_ENUM."MINIMIZE UI") -> ()  [unwired: 9 in, 2 out]
          }
        }
        n714 = local write "CAMERA ROI MAX TEMP"(TRUE ("CAMERA ROI MAX TEMP")) -> ()
      }
      frame "Test Setup" {
        n715 = local read "LIVE FEED MIN TEMP"() -> (w1095:bool)
        n716 = local read "CAMERA ROI MIN TEMP"() -> (w1093:bool)
        n717 = local write "LIVE FEED MAX TEMP"(TRUE ("LIVE FEED MAX TEMP")) -> ()
        n718 = case shown="True" w1095 {
          selector: w1095 -> [_ w1102]
          frame False {
          }
          frame True {
            n719 = Not(x=w1102) -> (.not. x?=w1101:bool)
            n720 = local write "LIVE FEED MIN TEMP"(w1101) -> ()
            n721 = call "CAMERA LIVE FEED FGV.vi"("Enum - Menu"=CAMERA_LIVE_FEED_ENUM."CAMERA MINIMIZE") -> ()  [unwired: 9 in, 2 out]
          }
        }
        n722 = case shown="True" w1093 {
          selector: w1093 -> [_ w1099]
          frame False {
          }
          frame True {
            n723 = Not(x=w1099) -> (.not. x?=w1098:bool)
            n724 = local write "CAMERA ROI MIN TEMP"(w1098) -> ()
            n725 = call "IMAGE ANALYSIS.vi"("Enum"=POST_ANALYSIS_ENUM."MINIMIZE UI") -> ()  [unwired: 9 in, 2 out]
          }
        }
        n726 = local write "CAMERA ROI MAX TEMP"(TRUE ("CAMERA ROI MAX TEMP")) -> ()
      }
      frame "Acquire" {
        n727 = local read "LIVE FEED MIN TEMP"() -> (w1105:bool)
        n728 = local write "LIVE FEED MAX TEMP"(TRUE ("LIVE FEED MAX TEMP")) -> ()
        n729 = local read "CAMERA ROI MIN TEMP"() -> (w1103:bool)
        n730 = case shown="True" w1105 {
          selector: w1105 -> [_ w1112]
          frame False {
          }
          frame True {
            n731 = Not(x=w1112) -> (.not. x?=w1111:bool)
            n732 = local write "LIVE FEED MIN TEMP"(w1111) -> ()
            n733 = call "CAMERA LIVE FEED FGV.vi"("Enum - Menu"=CAMERA_LIVE_FEED_ENUM."CAMERA MINIMIZE") -> ()  [unwired: 9 in, 2 out]
          }
        }
        n734 = case shown="True" w1103 {
          selector: w1103 -> [_ w1109]
          frame False {
          }
          frame True {
            n735 = Not(x=w1109) -> (.not. x?=w1108:bool)
            n736 = local write "CAMERA ROI MIN TEMP"(w1108) -> ()
            n737 = call "IMAGE ANALYSIS.vi"("Enum"=POST_ANALYSIS_ENUM."MINIMIZE UI") -> ()  [unwired: 9 in, 2 out]
          }
        }
        n738 = local write "CAMERA ROI MAX TEMP"(TRUE ("CAMERA ROI MAX TEMP")) -> ()
      }
      frame "Adv Scar" {
        n739 = local read "CAMERA ROI MIN TEMP"() -> (w1113:bool)
        n740 = case shown="True" "LIVE FEED MAX TEMP" {
          selector: "LIVE FEED MAX TEMP" -> [_ w1134]
          frame False {
          }
          frame True {
            n741 = Not(x=w1134) -> (.not. x?=w1133:bool)
            n742 = local write "LIVE FEED MAX TEMP"(w1133) -> ()
            n743 = call "CAMERA LIVE FEED FGV.vi"("Enum - Menu"=CAMERA_LIVE_FEED_ENUM."CAMERA RESTORE") -> ("error out"=w1124:errorcluster)  [unwired: 9 in, 1 out]
            n744 = Type Cast(type=30, x=0) -> (*(type *) &x=w1128:i32)
            n745 = Add(x=w1128, y=48) -> (x+y=w1129:i32)
            n746 = call "CAMERA LIVE FEED FGV.vi"("Enum - Menu"=CAMERA_LIVE_FEED_ENUM."CAMERA MODE SET", "error in (no error)"=w1124, "CAMERA MODE"=w1129) -> ("error out"=w1121:errorcluster)  [unwired: 7 in, 1 out]
            n747 = call "CAMERA LIVE FEED FGV.vi"("Enum - Menu"=CAMERA_LIVE_FEED_ENUM."CAMERA GRAY", "error in (no error)"=w1121) -> ("error out"=w1120:errorcluster)  [unwired: 8 in, 1 out]
            n748 = call "LIST FILE NAMES.vi"("error in (no error)"=w1120) -> ("error out"=w1130:errorcluster, "filenames"=w1131:string[])  [unwired: 9 in]
            n749 = property on="FILE 3" class="CmbBox"(error in=w1130, "Strings[]"=w1131) -> ()  [unwired: 1 in, 2 out]
          }
        }
        n750 = case shown="True" w1113 {
          selector: w1113 -> [_ w1119]
          frame False {
          }
          frame True {
            n751 = Not(x=w1119) -> (.not. x?=w1118:bool)
            n752 = local write "CAMERA ROI MIN TEMP"(w1118) -> ()
            n753 = call "IMAGE ANALYSIS.vi"("Enum"=POST_ANALYSIS_ENUM."MINIMIZE UI") -> ()  [unwired: 9 in, 2 out]
          }
        }
        n754 = local write "CAMERA ROI MAX TEMP"(TRUE ("CAMERA ROI MAX TEMP")) -> ()
        "LIVE FEED MIN TEMP" <- TRUE ("LIVE FEED MIN TEMP")
      }
      frame "Adv Scar Report" {
        n755 = local read "CAMERA ROI MAX TEMP"() -> (w1135:bool)
        n756 = local read "LIVE FEED MIN TEMP"() -> (w1137:bool)
        n757 = local write "LIVE FEED MAX TEMP"(TRUE ("LIVE FEED MAX TEMP")) -> ()
        n758 = case shown="True" w1137 {
          selector: w1137 -> [_ w1146]
          frame False {
          }
          frame True {
            n759 = Not(x=w1146) -> (.not. x?=w1145:bool)
            n760 = local write "LIVE FEED MIN TEMP"(w1145) -> ()
            n761 = call "CAMERA LIVE FEED FGV.vi"("Enum - Menu"=CAMERA_LIVE_FEED_ENUM."CAMERA MINIMIZE") -> ()  [unwired: 9 in, 2 out]
          }
        }
        n762 = case shown="True" w1135 {
          selector: w1135 -> [_ w1143]
          frame False {
          }
          frame True {
            n763 = Not(x=w1143) -> (.not. x?=w1141:bool)
            n764 = local write "CAMERA ROI MAX TEMP"(w1141) -> ()
            n765 = call "IMAGE ANALYSIS.vi"("Enum"=POST_ANALYSIS_ENUM."SHOW UI") -> ("error out"=w1140:errorcluster)  [unwired: 9 in, 1 out]
            n766 = call "LIST FILE NAMES.vi"("error in (no error)"=w1140) -> ("filenames"=w1139:string[])  [unwired: 9 in, 1 out]
            n767 = property on="Test File List :" class="CmbBox"("Strings[]"=w1139) -> ()  [unwired: 2 in, 2 out]
          }
        }
        n768 = local write "CAMERA ROI MIN TEMP"(TRUE ("CAMERA ROI MIN TEMP")) -> ()
      }
      frame "Compare Files" {
        n769 = local read "LIVE FEED MIN TEMP"() -> (w1149:bool)
        n770 = local write "LIVE FEED MAX TEMP"(TRUE ("LIVE FEED MAX TEMP")) -> ()
        n771 = local read "CAMERA ROI MIN TEMP"() -> (w1147:bool)
        n772 = case shown="True" w1149 {
          selector: w1149 -> [_ w1156]
          frame False {
          }
          frame True {
            n773 = Not(x=w1156) -> (.not. x?=w1155:bool)
            n774 = local write "LIVE FEED MIN TEMP"(w1155) -> ()
            n775 = call "CAMERA LIVE FEED FGV.vi"("Enum - Menu"=CAMERA_LIVE_FEED_ENUM."CAMERA MINIMIZE") -> ()  [unwired: 9 in, 2 out]
          }
        }
        n776 = case shown="True" w1147 {
          selector: w1147 -> [_ w1153]
          frame False {
          }
          frame True {
            n777 = Not(x=w1153) -> (.not. x?=w1152:bool)
            n778 = local write "CAMERA ROI MIN TEMP"(w1152) -> ()
            n779 = call "IMAGE ANALYSIS.vi"("Enum"=POST_ANALYSIS_ENUM."MINIMIZE UI") -> ()  [unwired: 9 in, 2 out]
          }
        }
        n780 = local write "CAMERA ROI MAX TEMP"(TRUE ("CAMERA ROI MAX TEMP")) -> ()
      }
      frame "About" {
        n781 = local read "LIVE FEED MIN TEMP"() -> (w1159:bool)
        n782 = local write "LIVE FEED MAX TEMP"(TRUE ("LIVE FEED MAX TEMP")) -> ()
        n783 = local read "CAMERA ROI MIN TEMP"() -> (w1158:bool)
        n784 = case shown="True" w1159 {
          selector: w1159 -> [_ w1166]
          frame False {
          }
          frame True {
            n785 = Not(x=w1166) -> (.not. x?=w1165:bool)
            n786 = local write "LIVE FEED MIN TEMP"(w1165) -> ()
            n787 = call "CAMERA LIVE FEED FGV.vi"("Enum - Menu"=CAMERA_LIVE_FEED_ENUM."CAMERA MINIMIZE") -> ()  [unwired: 9 in, 2 out]
          }
        }
        n788 = case shown="True" w1158 {
          selector: w1158 -> [_ w1163]
          frame False {
          }
          frame True {
            n789 = Not(x=w1163) -> (.not. x?=w1162:bool)
            n790 = local write "CAMERA ROI MIN TEMP"(w1162) -> ()
            n791 = call "IMAGE ANALYSIS.vi"("Enum"=POST_ANALYSIS_ENUM."MINIMIZE UI") -> ()  [unwired: 9 in, 2 out]
          }
        }
        n792 = local write "CAMERA ROI MAX TEMP"(TRUE ("CAMERA ROI MIN TEMP")) -> ()
      }
      frame "Advance" {
        n793 = local read "LIVE FEED MIN TEMP"() -> (w1169:bool)
        n794 = local write "LIVE FEED MAX TEMP"(TRUE ("LIVE FEED MAX TEMP")) -> ()
        n795 = local read "CAMERA ROI MIN TEMP"() -> (w1167:bool)
        n796 = case shown="True" w1169 {
          selector: w1169 -> [_ w1176]
          frame False {
          }
          frame True {
            n797 = Not(x=w1176) -> (.not. x?=w1175:bool)
            n798 = local write "LIVE FEED MIN TEMP"(w1175) -> ()
            n799 = call "CAMERA LIVE FEED FGV.vi"("Enum - Menu"=CAMERA_LIVE_FEED_ENUM."CAMERA MINIMIZE") -> ()  [unwired: 9 in, 2 out]
          }
        }
        n800 = local write "CAMERA ROI MAX TEMP"(TRUE ("CAMERA ROI MAX TEMP")) -> ()
        n801 = case shown="True" w1167 {
          selector: w1167 -> [_ w1173]
          frame False {
          }
          frame True {
            n802 = Not(x=w1173) -> (.not. x?=w1172:bool)
            n803 = local write "CAMERA ROI MIN TEMP"(w1172) -> ()
            n804 = call "IMAGE ANALYSIS.vi"("Enum"=POST_ANALYSIS_ENUM."MINIMIZE UI") -> ()  [unwired: 9 in, 2 out]
          }
        }
      }
      frame "Mooha" {
        n805 = local read "LIVE FEED MIN TEMP"() -> (w1179:bool)
        n806 = local write "LIVE FEED MAX TEMP"(TRUE ("LIVE FEED MAX TEMP")) -> ()
        n807 = local read "CAMERA ROI MIN TEMP"() -> (w1177:bool)
        n808 = case shown="True" w1179 {
          selector: w1179 -> [_ w1186]
          frame False {
          }
          frame True {
            n809 = Not(x=w1186) -> (.not. x?=w1185:bool)
            n810 = local write "LIVE FEED MIN TEMP"(w1185) -> ()
